vi "ACTIVATION_SA.vi"(8 "error in (no error)":errorcluster) -> (0 "error out":errorcluster, 3 "STATUS":bool)   [LabVIEW 2017]
uses:
  <vilib>/registry/registry.llb/Registry RtKey.ctl
  <vilib>/registry/registry.llb/Read Registry Value Simple STR.vi
panel:
  out "date/time string":string
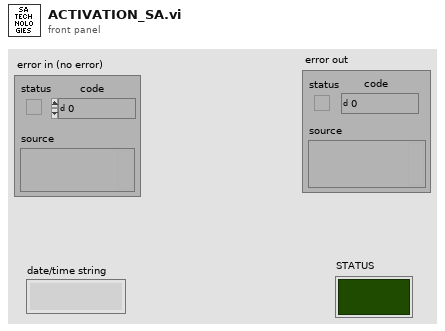
[diagram p1: front panel]
types:
  T1 = typedef "Registry RtKey.ctl" = enum32{"HKEY_CLASSES_ROOT", "HKEY_CURRENT_USER", "HKEY_LOCAL_MACHINE", "HKEY_USERS", "HKEY_PERFORMANCE_DATA", "HKEY_CURRENT_CONFIG", "HKEY_DYN_DATA"}
  T2 = typedef "Registry refnum.ctl" = refnum<k1>
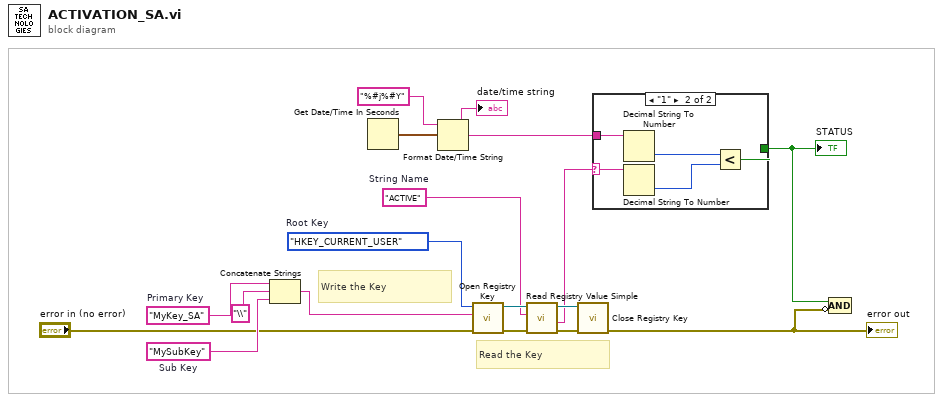
[diagram p0: block diagram]
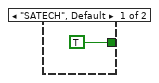
[diagram p2: hidden frame]
diagram:
  w11 = "MySubKey"  # Sub Key
  w9 = "MyKey_SA"  # Primary Key
  w10 = "ACTIVE"  # String Name
  w13 = Registry_RtKey."HKEY_CURRENT_USER"  # Root Key
  # "Read the Key"
  # "Write the Key"
  n1 = Concatenate Strings(w9, "\\", w11) -> (w12:string)
  n2 = Get Date/Time In Seconds() -> (seconds since 1Jan1904=w6:timestamp)
  n3 = Format Date/Time String(time format string (%c)="%#j%#Y", seconds (now)=w6) -> (date/time string=w3:string)  [unwired: 1 in]
  "date/time string" <- w3
  n4 = call <vilib>:"Open Registry Key.vi"("error in (no error)"="error in (no error)", "subkey"=w12, "root key (HKEY_LOCAL_MACHINE)"=w13) -> ("error out"=w14:errorcluster, "refnum out"=w15:T2)  [unwired: 7 in]
  n5 = call-poly <vilib>:"Read Registry Value Simple.vi"("error in (no error)"=w14, "value"=w10, "refnum"=w15) -> ("error out"=w17:errorcluster, "String/Binary data"=w4:string, "refnum out"=w16:T2)  [unwired: 3 in, 1 out]
  n6 = call <vilib>:"Close Registry Key.vi"("error in (no error)"=w17, "refnum"=w16) -> ("error out"=w1:errorcluster)  [unwired: 5 in]
  "error out" <- w1
  n7 = case shown="\"1\"" w4 {
    selector: w4 -> [_ w23]
    tunnel: [TRUE w19] -> w2
    tunnel: w3 -> [_ w22]
    frame "SATECH", Default {
    }
    frame "1" {
      n8 = Decimal String To Number(string=w22) -> (number=w21:i32)  [unwired: 2 in, 1 out]
      n9 = Decimal String To Number(string=w23) -> (number=w20:i32)  [unwired: 2 in, 1 out]
      n10 = Less?(x=w21, y=w20) -> (x < y?=w19:bool)
    }
  }
  "STATUS" <- w2
  n11 = Compound Arithmetic op=AND(w2, invert w1) -> ()  [unwired: 1 out]
